vi "bool_to_64.vi"(2 "N":i32, 3 "IN":bool[](array[boolean])) -> (1 "N64":u64 format="%b")   [LabVIEW 2019, in "Logik.lvlib"]
uses:
  Logik.lvlib
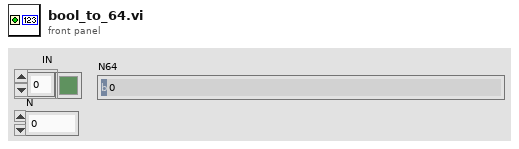
[diagram p1: front panel]
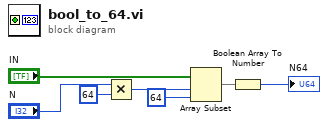
[diagram p0: block diagram]
diagram:
  n1 = Multiply(x="N", y=64 ("length")) -> (x*y=w1:i32)
  n2 = Array Subset(array="IN", index=w1, length=64) -> (w7:bool[])
  n3 = Boolean Array To Number(Boolean array=w7) -> (number=→"N64":u64)
